vi "gjsonParser.vi"(11 "StringToParse":string) -> (3 "ParsedString":string)   [LabVIEW 2015, in "Json2Labv.lvlib"]
uses:
  Json2Labv.lvlib
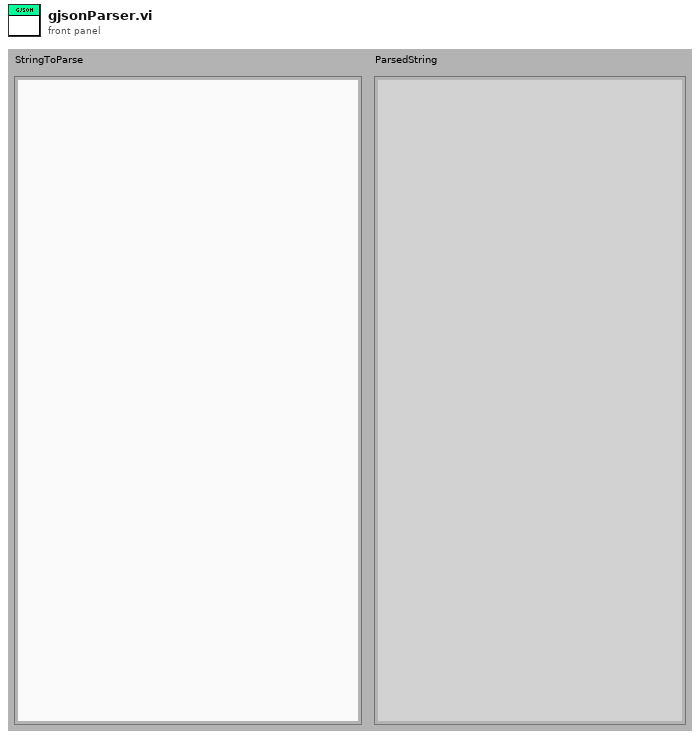
[diagram p1: front panel]
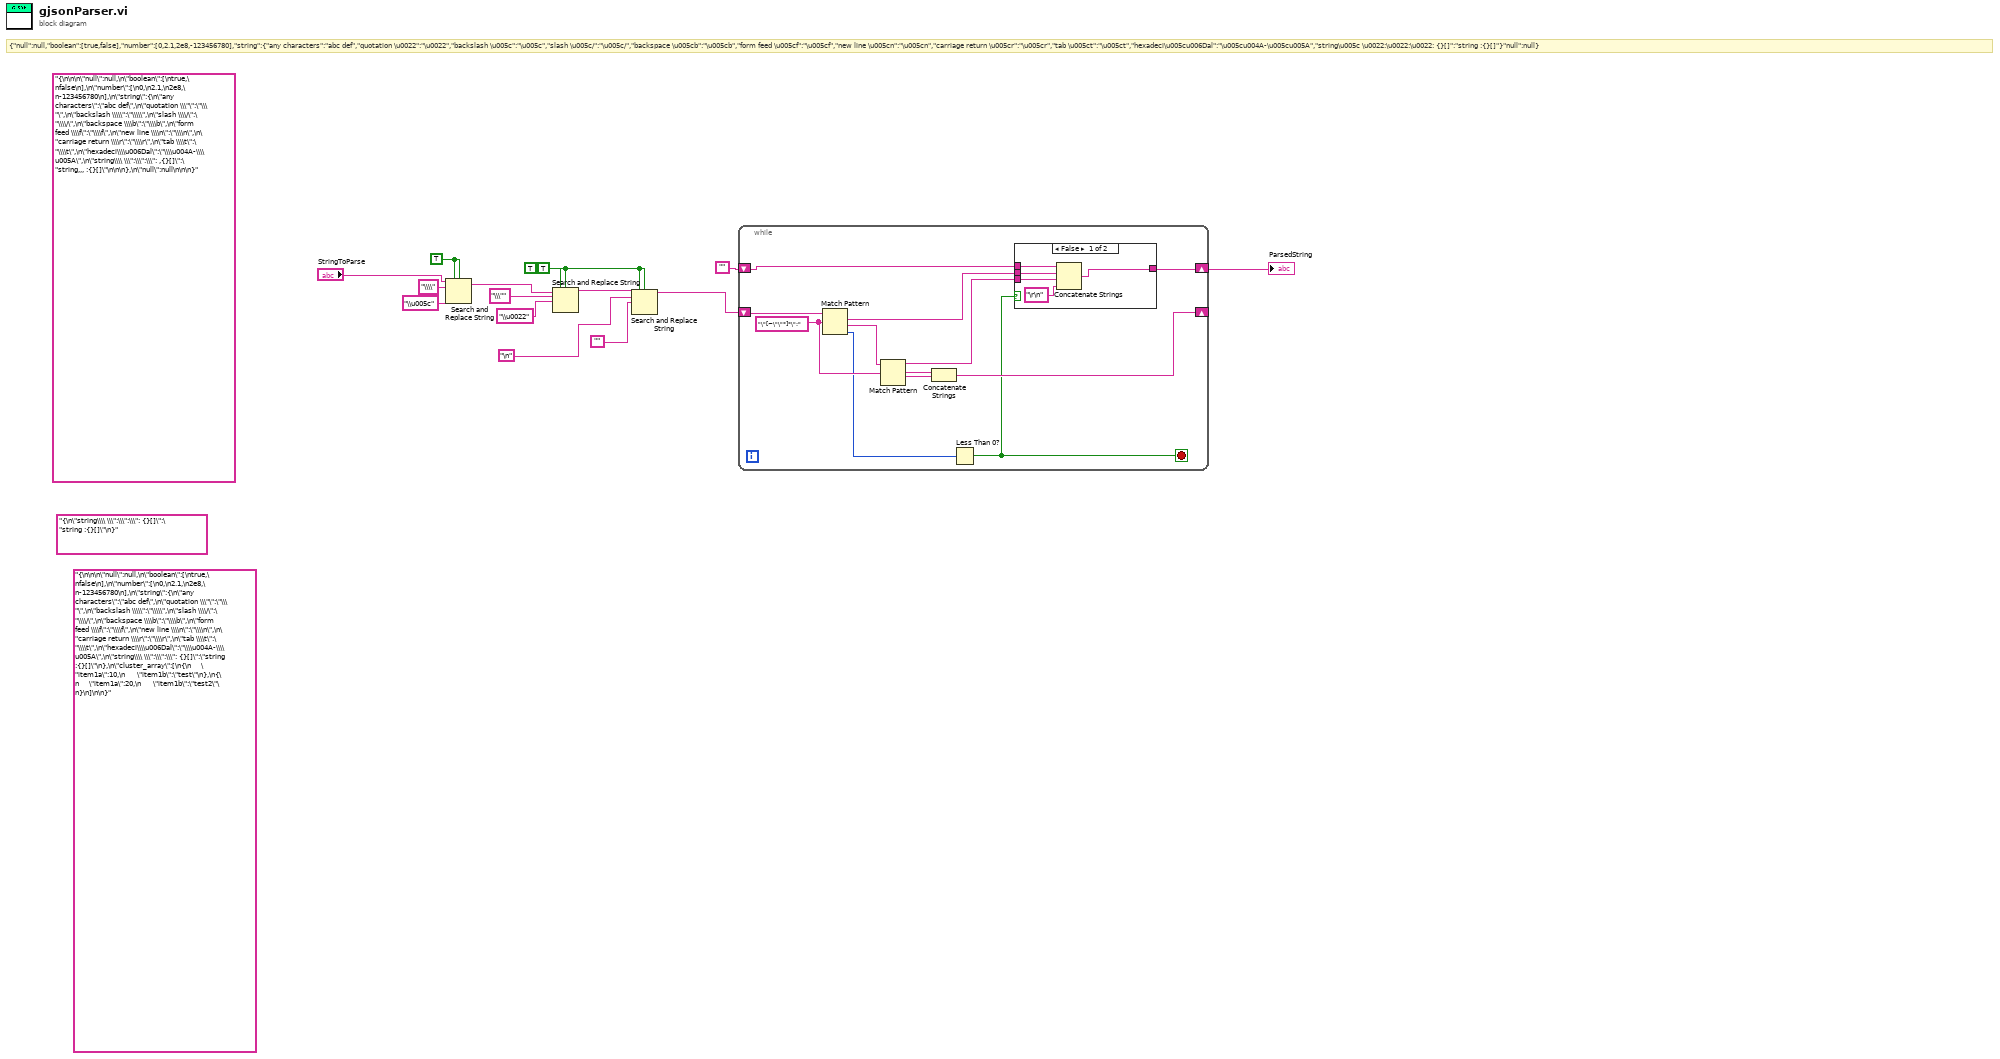
[diagram p0: block diagram]
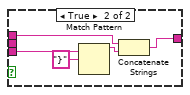
[diagram p2: hidden frame]
diagram:
  (unwired) "{\n\n\n\"null\":null,\n\"boolean\":[\ntrue,\nfalse\n],\n\"number\":[\n0,\n2.1,\n2e8,\n-123456780\n],\n\"string\":{\n\"any characters\":\"abc def\",\n\"quotation \\\"\":\"\\\"\",\n\"backslash \\\\\":\"\\\\\",\n\"slash \\\\/\":\"\\\\/\",\n\"backspace \\\\b\":\"\\\\b\",\n\"form feed \\\\f\":\"\\\\f\",\n\"new line \\\\n\":\"\\\\n\",\n\"carriage return \\\\r\":\"\\\\r\",\n\"tab \\\\t\":\"\\\\t\",\n\"hexadeci\\\\u006Dal\":\"\\\\u004A-\\\\u005A\",\n\"string\\\\ \\\":\\\":\\\": {}[]\":\"string :{}[]\"\n},\n\"cluster_array\":[\n{\n     \"item1a\":10,\n      \"item1b\":\"test\"\n},\n{\n     \"item1a\":20,\n      \"item1b\":\"test2\"\n}\n]\n\n}"
  (unwired) "{\n\"string\\\\ \\\":\\\":\\\": {}[]\":\"string :{}[]\"\n}"
  w11 = TRUE ("ignore case? (F)")
  w6 = TRUE ("ignore case? (F)")
  (unwired) "{\n\n\n\"null\":null,\n\"boolean\":[\ntrue,\nfalse\n],\n\"number\":[\n0,\n2.1,\n2e8,\n-123456780\n],\n\"string\":{\n\"any characters\":\"abc def\",\n\"quotation \\\"\":\"\\\"\",\n\"backslash \\\\\":\"\\\\\",\n\"slash \\\\/\":\"\\\\/\",\n\"backspace \\\\b\":\"\\\\b\",\n\"form feed \\\\f\":\"\\\\f\",\n\"new line \\\\n\":\"\\\\n\",\n\"carriage return \\\\r\":\"\\\\r\",\n\"tab \\\\t\":\"\\\\t\",\n\"hexadeci\\\\u006Dal\":\"\\\\u004A-\\\\u005A\",\n\"string\\\\ \\\":\\\":\\\": ,{}[]\":\"string,,, :{}[]\"\n\n\n},\n\"null\":null\n\n\n}"
  # "{\"null\":null,\"boolean\":[true,false],\"number\":[0,2.1,2e8,-123456780],\"string\":{\"any characters\":\"abc def\",\"quotation \\u0022\":\"\\u0022\",\"backslash \\u005c\":\"\\u005c\",\"slash \\u005c/\":\"\\u005c/\",\"backspace \\u005cb\":\"\\u005cb\",\"form feed \\u005cf\":\"\\u005cf\",\"new line \\u005cn\":\"\\u005cn\",\"carriage return \\u005cr\":\"\\u005cr\",\"tab \\u005ct\":\"\\u005ct\",\"hexadeci\\u005cu006Dal\":\"\\u005cu004A-\\u005cu005A\",\"string\\u005c \\u0022:\\u0022:\\u0022: {}[]\":\"string :{}[]\"}\"null\":null}"
  n1 = Search and Replace String(replace all?=w11, case sensitive?=w11, input string="StringToParse", search string="\\\\", replace string="\\u005c" ("replace string (\"\")")) -> (result string=w9:string)  [unwired: 3 in, 3 out]
  n2 = Search and Replace String(replace all?=TRUE ("replace all? (F)"), case sensitive?=w6, input string=w9, search string="\\\"", replace string="\\u0022" ("replace string (\"\")")) -> (result string=w8:string)  [unwired: 3 in, 3 out]
  n3 = Search and Replace String(replace all?=w6, case sensitive?=w6, input string=w8, search string="\n", replace string="") -> (result string=w2:string)  [unwired: 3 in, 3 out]
  n4 = while {
    shift-right: [w18] -> _
    shift-left: w2 -> [w27]
    shift-right: [w26] -> w3
    shift-left: "" -> [w25]
    stop <- w16 stop-if-true
    w22 = "\"[~\"\"*]*\":" ("regular expression")
    n5 = Match Pattern(string=w27, regular expression=w22) -> (match substring=w24:string, after substring=w23:string, offset past match=w17:i32)  [unwired: 1 in, 1 out]
    n6 = Match Pattern(string=w23, regular expression=w22) -> (before substring=w21:string, match substring=w19:string, after substring=w20:string)  [unwired: 1 in, 1 out]
    n7 = Concatenate Strings(w19, w20) -> (w18:string)
    n8 = Less Than 0?(x=w17) -> (x < 0?=w16:bool)
    n9 = case shown="False" w16 {
      tunnel: [w32 w33] -> w26
      tunnel: w25 -> [w31 w34]
      tunnel: w24 -> [w30 _]
      tunnel: w21 -> [w28 w37]
      frame False {
        n10 = Concatenate Strings(w31, w30, w28, "\r\n" ("string")) -> (w32:string)
      }
      frame True {
        n11 = Match Pattern(string=w37, regular expression="}") -> (before substring=w35:string)  [unwired: 1 in, 3 out]
        n12 = Concatenate Strings(w34, w35) -> (w33:string)
      }
    }
  }
  "ParsedString" <- w3
